vi "Build Test Result.vi"(8 "error in (no error)":errorcluster, 10 "Result Data":T1, 11 "Test Result in":refnum<class "Test Result.lvclass">) -> (0 "error out":errorcluster, 3 "Test Result out":refnum<class "Test Result.lvclass">)   [LabVIEW 2021, in "Sequence Engine.lvlib" / "Test Result.lvclass"]
uses:
  Test Result.lvclass
  Result Data.ctl
  Test Status.ctl
  Test Result.lvclass/Test Result.ctl
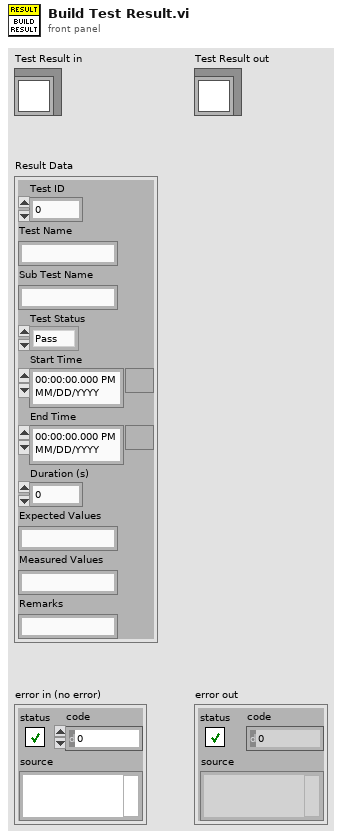
[diagram p1: front panel]
types:
  T1 = typedef "Sequence Engine.lvlib/Test Result.lvclass/Result Data.ctl" = cluster{"Test ID":u32, "Test Name":string, "Sub Test Name":string, "Test Status":T2, "Start Time":timestamp, "End Time":timestamp, "Duration (s)":dbl, "Expected Values":string, "Measured Values":string, "Remarks":string}
  T2 = typedef "Sequence Engine.lvlib/Test Result.lvclass/Test Status.ctl" = enum16{"Pass", "Fail", "Aborted", "Skipped"}
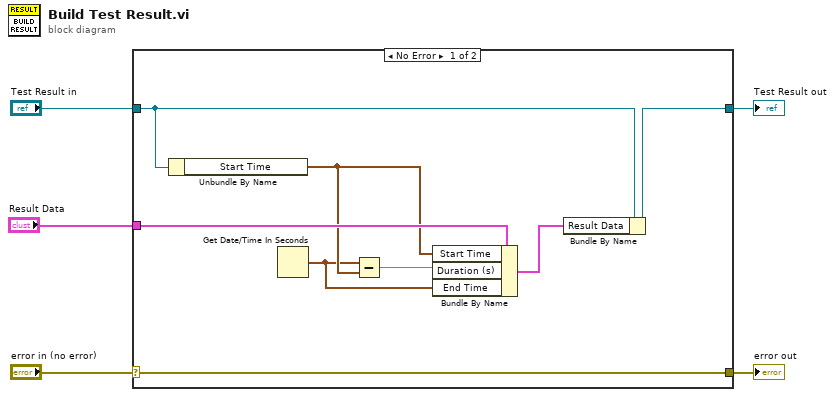
[diagram p0: block diagram]
diagram:
  n1 = case shown="No Error" "error in (no error)" {
    selector: "error in (no error)" -> [w13 w15]
    tunnel: [w13 w15] -> w4
    tunnel: [w11 w14] -> w2
    tunnel: "Test Result in" -> [w12 w14]
    tunnel: "Result Data" -> [w9 _]
    frame No Error {
      n2 = Unbundle By Name(w12) -> ("Start Time"=w8:timestamp)
      n3 = Get Date/Time In Seconds() -> (seconds since 1Jan1904=w6:timestamp)
      n4 = Subtract(x=w6, y=w8) -> (x-y=w7:dbl)
      n5 = Bundle By Name(cluster=w9, "Start Time"=w8, "Duration (s)"=w7, "End Time"=w6) -> (w10:T1)
      n6 = Bundle By Name(cluster=w12, "Result Data"=w10) -> (w11:refnum<class "Test Result.lvclass">)
    }
    frame Error {
    }
  }
  "error out" <- w4
  "Test Result out" <- w2
